vi "HumanActionCache.vi"(4 "Enable Field Oriented Drive":bool, 5 "AutoSpeakerAngle":dbl, 6 "State":i32, 7 "Rotation":dbl, 8 "Right X":dbl, 9 "Right Y":dbl, 10 "Left X":dbl, 11 "Left Y":dbl) -> (1 "AMotorDemand":dbl, 2 "YMotorDemand":dbl, 3 "XMotorDemand":dbl)   [LabVIEW 2023]
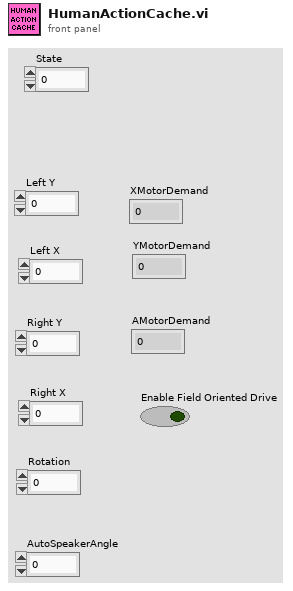
[diagram p1: front panel]
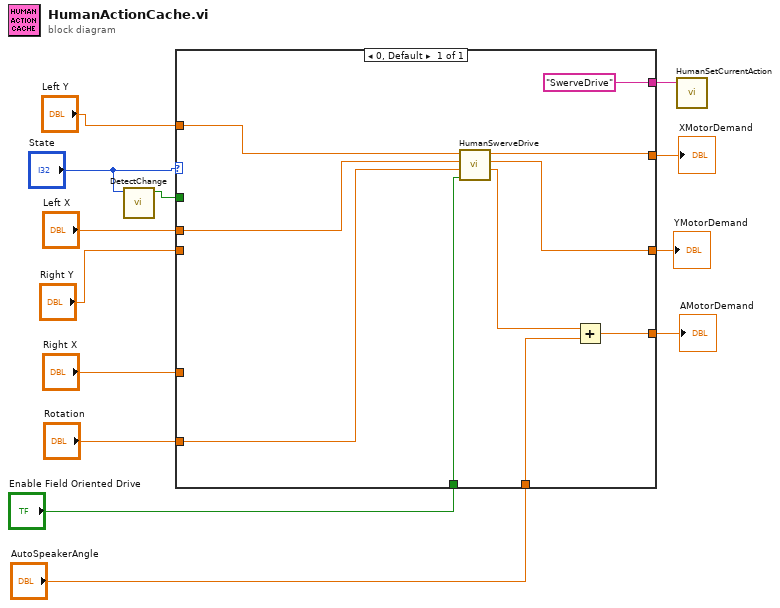
[diagram p0: block diagram]
diagram:
  n1 = call "DetectChange.vi"("Value"="State") -> ("Changed"=w7:bool)  [unwired: 10 in]
  n2 = case shown="0, Default" "State" {
    tunnel: "Left Y" -> [w22]
    tunnel: "Right X" -> [_]
    tunnel: [w19] -> w11
    tunnel: [w18] -> w10
    tunnel: "Right Y" -> [_]
    tunnel: w7 -> [_]
    tunnel: ["SwerveDrive"] -> w6
    tunnel: "Left X" -> [w21]
    tunnel: "Rotation" -> [w20]
    tunnel: [w14] -> w3
    tunnel: "Enable Field Oriented Drive" -> [w17]
    tunnel: "AutoSpeakerAngle" -> [w16]
    frame 0, Default {
      n3 = call "HumanSwerveDrive.vi"("Enable Field Oriented Drive"=w17, "Rotation"=w20, "Y"=w21, "X"=w22) -> ("A"=w15:dbl, "Y"=w18:dbl, "X"=w19:dbl)  [unwired: 5 in]
      n4 = Add(x=w15, y=w16) -> (x+y=w14:dbl)
    }
  }
  "XMotorDemand" <- w11
  "YMotorDemand" <- w10
  "AMotorDemand" <- w3
  n5 = call "HumanSetCurrentAction.vi"("CurrentState"=w6) -> ()  [unwired: 11 in]
